vi "AssertValueByFocusTag.vi"(0 "VI Reference In":refnum<vi>, 1 "Test Label":string, 2 "delimiter (>>)":string=">>", 3 "Assert Only? (F)":bool, 5 "Control Path":string, 7 "Focus Item Tag":string, 11 "Error In":errorcluster, 12 "Assert Interval(10 ms)":u32=10, 13 "Timeout(5 sec)":dbl=5.0) -> (4 "VI Reference Out":refnum<vi>, 6 "Asserted Value":string, 15 "Error Out":errorcluster)   [LabVIEW 2016, in "Drona.lvlib" / "AssertControlValue.lvlib" / "AssertTree.lvlib"]
doc: "Asserts if the focus item tag for the tree control is equal.\n\nThe input control name is given as a string , incase of path, use delimiters inbetween the path.\nThis VI gets the value of the control, untill the value is equal to the input value."
uses:
  AssertTree.lvlib
  Get/GetControlRef/GetControlRefByPath.vi
  <vilib>/addons/_JKI Toolkits/Caraya/classes/Assert/Assert Equal Value_Variant.vi
  <vilib>/addons/_JKI Toolkits/Caraya/classes/Assert/Assert.lvclass
  Get/GetControlRef/GetControlRef.lvlib
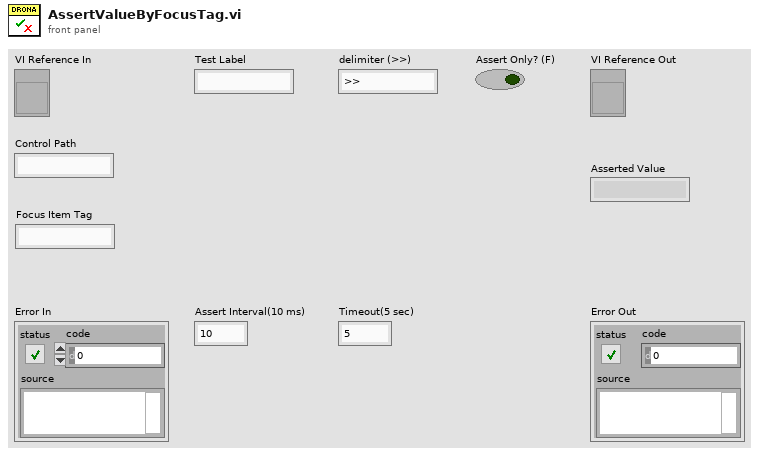
[diagram p1: front panel]
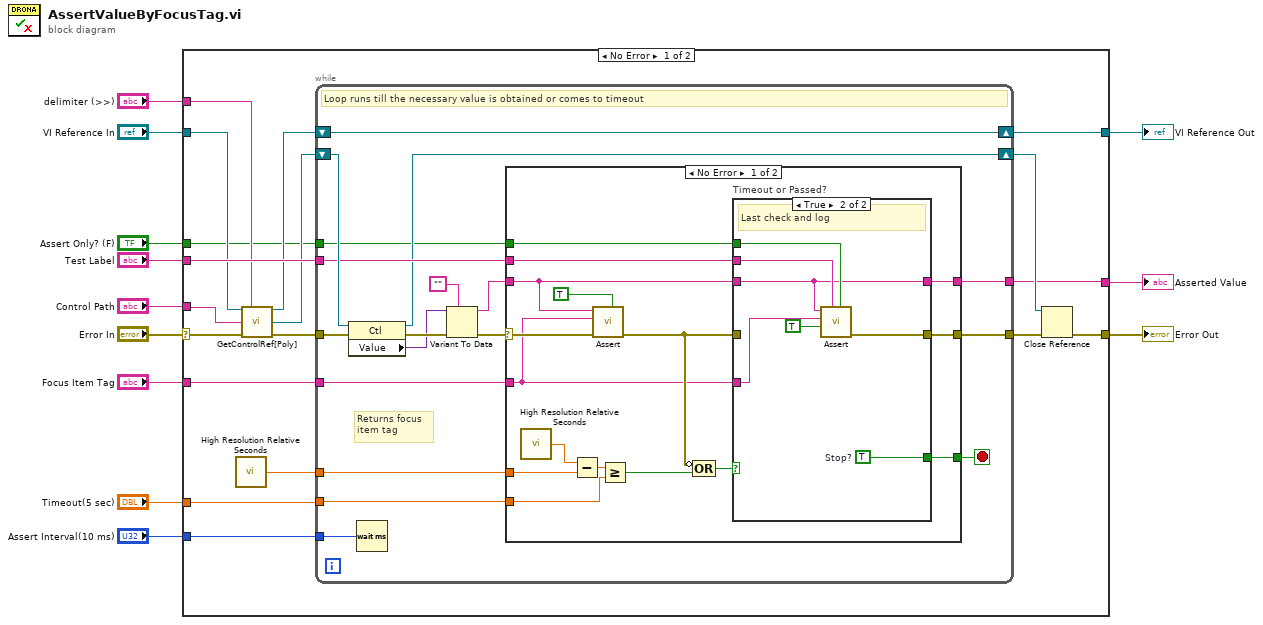
[diagram p0: block diagram]
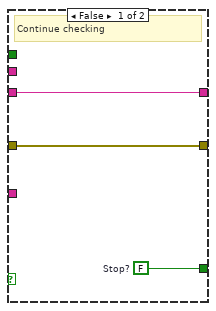
[diagram p2: hidden frame]
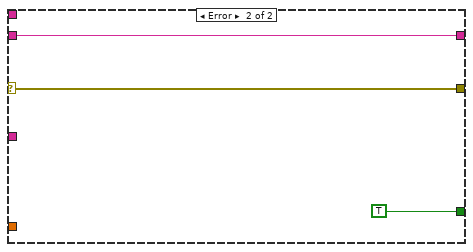
[diagram p3: hidden frame]
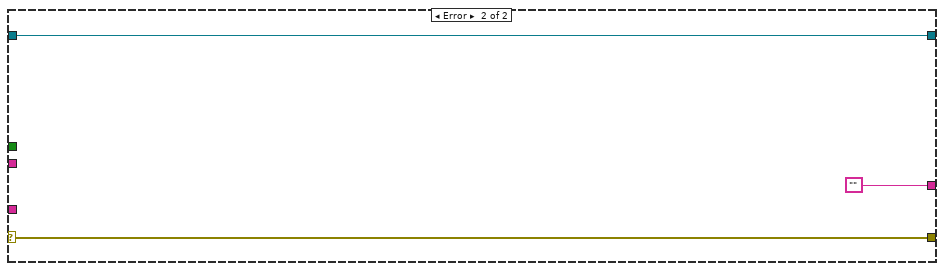
[diagram p4: hidden frame]
diagram:
  n1 = case shown="No Error" "Error In" {
    selector: "Error In" -> [w24 w80]
    tunnel: "Timeout(5 sec)" -> [w30 _]
    tunnel: [w29 w79] -> w11
    tunnel: "Focus Item Tag" -> [w28 _]
    tunnel: [w17 w80] -> w9
    tunnel: "Assert Interval(10 ms)" -> [w26 _]
    tunnel: "Test Label" -> [w25 _]
    tunnel: "VI Reference In" -> [w23 w79]
    tunnel: "Control Path" -> [w22 _]
    tunnel: "delimiter (>>)" -> [w15 _]
    tunnel: "Assert Only? (F)" -> [w14 _]
    tunnel: [w13 ""] -> w1
    frame No Error {
      n2 = call <vilib>:"High Resolution Relative Seconds.vi"() -> ("relative seconds"=w21:dbl)
      n3 = call-poly "GetControlRef[Poly].vi"("VI Reference In"=w23, "delimiter (>>)"=w15, "Control Path"=w22, "error In"=w24) -> ("VI Reference Out"=w19:refnum<vi>, "Ctl Refnum"=w18:refnum<vi>, "error out"=w20:errorcluster)  [unwired: 9 in]
      n4 = while {
        tunnel: w28 -> [w42]
        tunnel: w30 -> [w47]
        tunnel: w21 -> [w48]
        tunnel: w20 -> [w41]
        tunnel: [w45] -> w27
        tunnel: w26 -> [w43]
        tunnel: w25 -> [w38]
        shift-right: [w39] -> w29
        shift-left: w19 -> [w39]
        shift-right: [w37] -> w16
        shift-left: w18 -> [w40]
        tunnel: w14 -> [w36]
        tunnel: [w35] -> w13
        stop <- w46 stop-if-true
        # "Returns focus \nitem tag"
        # "Loop runs till the necessary value is obtained or comes to timeout"
        n5 = property on="Property Node" class="Ctl"(reference=w40, error in=w41) -> (reference out=w37:refnum<vi>, error out=w44:errorcluster, "Value"=w32:variant)
        n6 = Wait (ms)(milliseconds to wait=w43) -> ()  [unwired: 1 out]
        n7 = Variant To Data(error in=w44, type="", Variant=w32) -> (data=w31:string, error out=w34:errorcluster)
        n8 = case shown="No Error" w34 {
          selector: w34 -> [w60 w77]
          tunnel: w48 -> [w64 _]
          tunnel: w47 -> [w61 _]
          tunnel: [w51 TRUE] -> w46
          tunnel: [w52 w77] -> w45
          tunnel: w42 -> [w53 _]
          tunnel: w31 -> [w54 w75]
          tunnel: w38 -> [w59 _]
          tunnel: w36 -> [w50 _]
          tunnel: [w49 w75] -> w35
          frame No Error {
            n9 = call <vilib>:"High Resolution Relative Seconds.vi"() -> ("relative seconds"=w63:dbl)
            n10 = Subtract(x=w63, y=w64) -> (x-y=w62:dbl)
            n11 = call-poly <vilib>:"Assert.vi"("Assert Only? (F)"=TRUE, "error in (no error)"=w60, "Y"=w53, "X"=w54) -> ("error out"=w57:errorcluster)  [unwired: 6 in, 1 out]
            n12 = Greater Or Equal?(x=w62, y=w61) -> (x >= y?=w58:bool)
            n13 = Compound Arithmetic op=OR(invert w57, w58) -> (w56:bool)
            n14 = case "Timeout or Passed?" shown="True" w56 {
              tunnel: w57 -> [w67 _]
              tunnel: w53 -> [_ w73]
              tunnel: w54 -> [w65 w68]
              tunnel: w59 -> [_ w74]
              tunnel: [w67 w72] -> w52
              tunnel: [w66 w71] -> w51
              tunnel: w50 -> [_ w69]
              tunnel: [w65 w68] -> w49
              frame False {
                w66 = FALSE  # Stop?
                # "Continue checking"
              }
              frame True {
                w71 = TRUE  # Stop?
                # "Last check and log"
                n15 = call-poly <vilib>:"Assert.vi"("Assert Only? (F)"=w69, "Label"=w74, "Register with caller test (F)"=TRUE, "Y"=w73, "X"=w68) -> ("error out"=w72:errorcluster)  [unwired: 5 in, 1 out]
              }
            }
          }
          frame Error {
          }
        }
      }
      n16 = Close Reference(reference=w16, error in (no error)=w27) -> (error out=w17:errorcluster)
    }
    frame Error {
    }
  }
  "Error Out" <- w9
  "VI Reference Out" <- w11
  "Asserted Value" <- w1
